vi "Actor Core.vi"(8 "error in":errorcluster, 11 "Nested in":refnum<class "UI Actor.lvclass">) -> (0 "error out":errorcluster, 3 "Actor out":refnum<class "Actor.lvclass">)   [LabVIEW 2020, in "UI Actor.lvlib" / "UI Actor.lvclass"]
doc: "Override de Actor Core, nos sirve para crear una interfaz amigable con el usuario."
uses:
  UI Actor.lvclass
  C:/Program Files/National Instruments/LabVIEW 2020/vi.lib/ActorFramework/Actor/Actor.lvclass
  <vilib>/ActorFramework/Actor/Actor.lvclass
  <vilib>/ActorFramework/Actor/Actor.lvclass/Actor.ctl
  <vilib>/ActorFramework/Message Enqueuer/Message Enqueuer.lvclass/Message Enqueuer.ctl
  UI Actor.lvclass/UI Actor.ctl
  <vilib>/ActorFramework/Message Enqueuer/Init from Existing Queue.vi
  <vilib>/ActorFramework/Message Enqueuer/Enqueue.vi
  UI Actor Messages/Close VISA Msg/Close VISA Msg.lvclass
  C:/Program Files/National Instruments/LabVIEW 2020/vi.lib/ActorFramework/Message/Message.lvclass
  <vilib>/ActorFramework/Stop Msg/Stop Msg.lvclass
  <vilib>/ActorFramework/Message Priority Queue/Priority Enqueue.vi
  <vilib>/ActorFramework/Message Enqueuer/Message Enqueuer.lvclass
  Abstract/Serial Device/Serial Device.lvclass
panel:
  out "String":string
  in  "Channel":u8
  out "Distancia":i32(slide) scale=0.0..200.0
  in  "CANAL2":bool
  in  "CANAL1 3":bool
  in  "Pin Number":u8
  in  "Set Pin":bool
  in  "CANAL1 2":bool
  in  "Set Port":bool[](array[boolean])
  in  "CANAL1 5":bool
  in  "Pin Number":u8
  out "Read Pin":bool
  in  "CANAL1 4":bool
  out "Read Port":bool[](array[boolean])
  # "Pin del 1 al 4"
  # "MSB"
  # "LSB"
  # "Pin del 1 al 4"
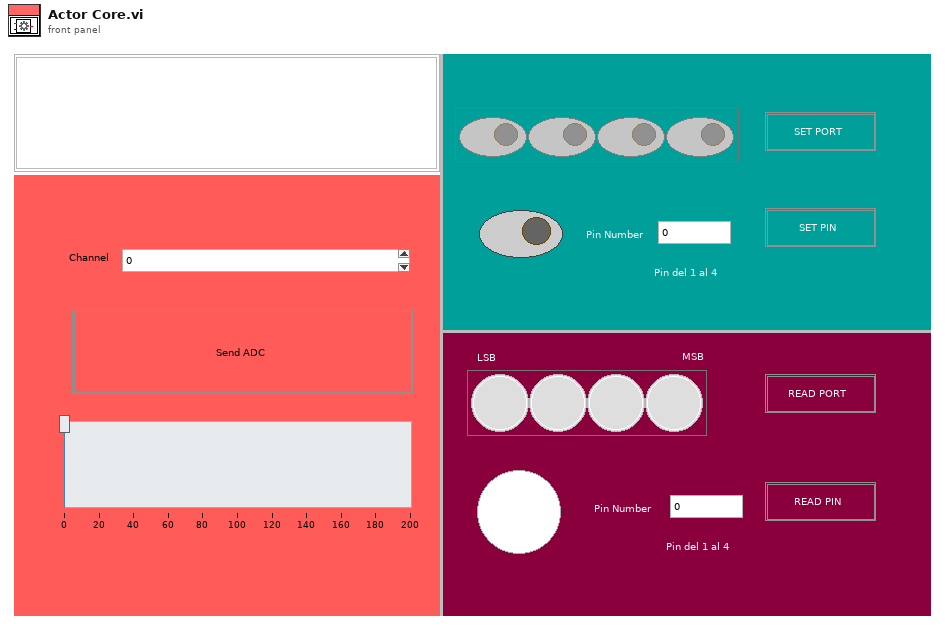
[diagram p1: front panel]
types:
  T1 = cluster{"Stop":refnum<user-event>, "LIGHT":refnum<user-event>, "Distancia":refnum<user-event>, "Read Port":refnum<user-event>, "Read Pin":refnum<user-event>, "String":refnum<user-event>}
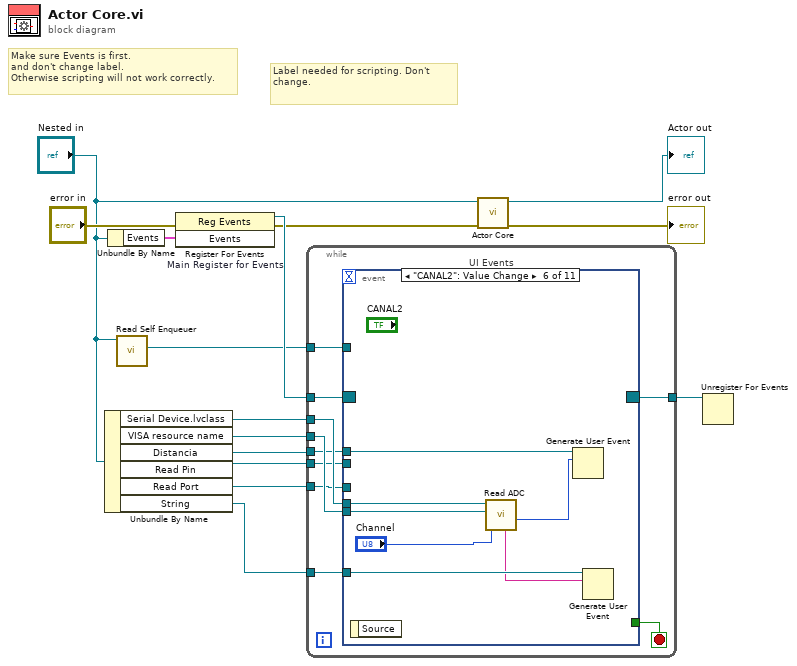
[diagram p0: block diagram]
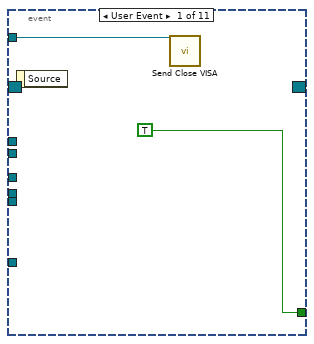
[diagram p2: hidden frame]
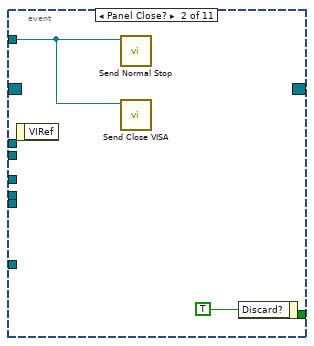
[diagram p3: hidden frame]
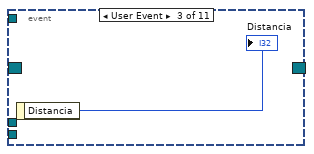
[diagram p4: hidden frame]
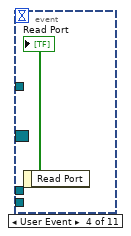
[diagram p5: hidden frame]
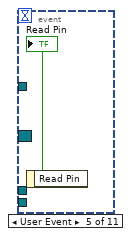
[diagram p6: hidden frame]
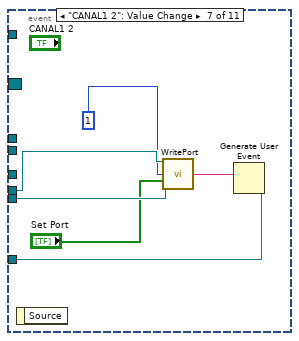
[diagram p7: hidden frame]
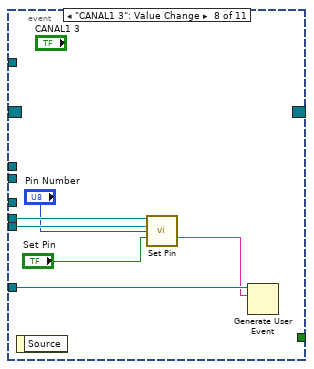
[diagram p8: hidden frame]
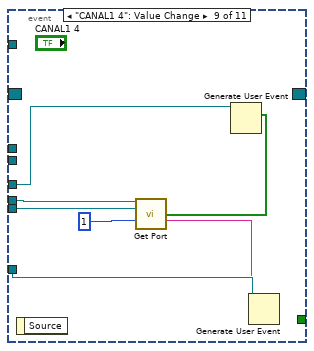
[diagram p9: hidden frame]
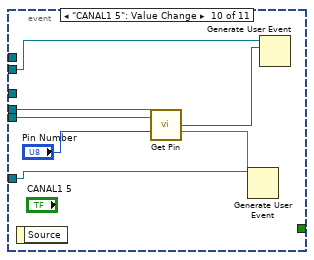
[diagram p10: hidden frame]
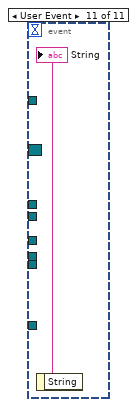
[diagram p11: hidden frame]
diagram:
  # "Label needed for scripting. Don't change."
  # "Make sure Events is first.\nand don't change label.\nOtherwise scripting will not work correctly."
  n1 = Unbundle By Name("Nested in") -> ("Serial Device.lvclass"=w6:refnum<class "Serial Device.lvclass">, "VISA resource name"=w5:refnum<visa-resource-name>, "Distancia"=w4:refnum<user-event>, "Read Pin"=w2:refnum<user-event>, "Read Port"=w3:refnum<user-event>, "String"=w1:refnum<user-event>)
  n2 = Unbundle By Name("Nested in") -> ("Events"=w12:T1)
  n3 = call <vilib>:"Read Self Enqueuer.vi"("Actor"="Nested in") -> ("Self Enqueuer"=w10:refnum<class "Message Enqueuer.lvclass">)  [unwired: 10 in]
  n4 = register-events "Main Register for Events"(error in="error in", w12) -> (reference out=w13:refnum<event-registration>, error out=w8:errorcluster)  [unwired: 1 in]
  n5 = while {
    tunnel: w13 -> [w25]
    tunnel: [w23] -> w11
    tunnel: w10 -> [w22]
    tunnel: w6 -> [w21]
    tunnel: w5 -> [w20]
    tunnel: w4 -> [w19]
    tunnel: w1 -> [w18]
    tunnel: w3 -> [w17]
    tunnel: w2 -> [w16]
    stop <- w24 stop-if-true
    n6 = event "UI Events" shown="[5] \"CANAL2\": Value Change" {
      selector: w25 -> [_ _ _ _ _ _ _ _ _ _ _]
      dyn-events: [_ _ _ _ _ _ _ _ _ _ _] -> w23
      timeout: _ -> [_ _ _ _ _ _ _ _ _ _ _]
      tunnel: [TRUE _ _ _ _ _ _ _ _ _ _] -> w24
      tunnel: w22 -> [w26 w28 _ _ _ _ _ _ _ _ _]
      tunnel: w21 -> [_ _ _ _ _ w39 w45 w51 w58 w65 _]
      tunnel: w20 -> [_ _ _ _ _ w38 w44 w50 w57 w64 _]
      tunnel: w19 -> [_ _ _ _ _ w36 _ _ _ _ _]
      tunnel: w18 -> [_ _ _ _ _ w34 w42 w47 w53 w60 _]
      tunnel: w17 -> [_ _ _ _ _ _ _ _ w55 _ _]
      tunnel: w16 -> [_ _ _ _ _ _ _ _ _ w62 _]
      event User Event {
        n7 = event-data() -> ()  [unwired: 1 in, 1 out]
        n8 = call "Send Close VISA.vi"("Message Enqueuer"=w26) -> ()  [unwired: 9 in, 2 out]
      }
      event Panel Close? {
        n9 = event-data() -> ()  [unwired: 1 in, 1 out]
        n10 = call <vilib>:"Send Normal Stop.vi"("Message Enqueuer"=w28) -> ()  [unwired: 10 in, 1 out]
        n11 = call "Send Close VISA.vi"("Message Enqueuer"=w28) -> ()  [unwired: 9 in, 2 out]
        n12 = event-data("Discard?"=TRUE) -> ()  [unwired: 1 in, 1 out]
      }
      event User Event {
        n13 = event-data() -> ("Distancia"=→"Distancia":i32)  [unwired: 1 in]
      }
      event User Event {
        n14 = event-data() -> ("Read Port"=→"Read Port":bool[])  [unwired: 1 in]
      }
      event User Event {
        n15 = event-data() -> ("Read Pin"=→"Read Pin":bool)  [unwired: 1 in]
      }
      event "CANAL2": Value Change {
        n16 = event-data() -> ()  [unwired: 1 in, 1 out]
        n17 = call-dynamic "Read ADC.vi"("Canal"="Channel", "VISA resource name"=w38, "Serial Device in"=w39) -> ("Response"=w35:i32, "String"=w33:string)  [unwired: 4 in, 3 out]
        n18 = Generate User Event(user event=w36, event data cluster=w35) -> ()  [unwired: 2 in, 2 out]
        n19 = Generate User Event(user event=w34, event data cluster=w33) -> ()  [unwired: 2 in, 2 out]
      }
      event "CANAL1 2": Value Change {
        n20 = event-data() -> ()  [unwired: 1 in, 1 out]
        n21 = call-dynamic "WritePort.vi"("Serial Device in"=w45, "VISA resource name"=w44, "Puerto"=u8 1, "Array"="Set Port") -> ("Expected response"=w41:string)  [unwired: 8 in, 3 out]
        n22 = Generate User Event(user event=w42, event data cluster=w41) -> ()  [unwired: 2 in, 2 out]
      }
      event "CANAL1 3": Value Change {
        n23 = event-data() -> ()  [unwired: 1 in, 1 out]
        n24 = call-dynamic "Set Pin.vi"("Serial Device in"=w51, "VISA resource name"=w50, "Pin"="Pin Number", "Pin State"="Set Pin") -> ("Response"=w46:string)  [unwired: 8 in, 3 out]
        n25 = Generate User Event(user event=w47, event data cluster=w46) -> ()  [unwired: 2 in, 2 out]
      }
      event "CANAL1 4": Value Change {
        n26 = event-data() -> ()  [unwired: 1 in, 1 out]
        n27 = call-dynamic "Get Port.vi"("Serial Device in"=w58, "VISA resource name"=w57, "Puerto"=u8 1) -> ("bool response"=w54:bool[], "Response"=w52:string)  [unwired: 8 in, 3 out]
        n28 = Generate User Event(user event=w55, event data cluster=w54) -> ()  [unwired: 2 in, 2 out]
        n29 = Generate User Event(user event=w53, event data cluster=w52) -> ()  [unwired: 2 in, 2 out]
      }
      event "CANAL1 5": Value Change {
        n30 = event-data() -> ()  [unwired: 1 in, 1 out]
        n31 = call-dynamic "Get Pin.vi"("Serial Device in"=w65, "VISA resource name"=w64, "Pin"="Pin Number") -> ("Boolean"=w61:bool, "Response"=w59:string)  [unwired: 8 in, 3 out]
        n32 = Generate User Event(user event=w60, event data cluster=w59) -> ()  [unwired: 2 in, 2 out]
        n33 = Generate User Event(user event=w62, event data cluster=w61) -> ()  [unwired: 2 in, 2 out]
      }
      event User Event {
        n34 = event-data() -> ("String"=→"String":string)  [unwired: 1 in]
      }
    }
  }
  n35 = call-parent "Actor Core.vi"("error in"=w8, "Actor in"="Nested in") -> ("error out"=→"error out":errorcluster, "Actor out"=→"Actor out":refnum<class "Actor.lvclass">)  [unwired: 8 in]
  n36 = Unregister For Events(event registration refnum=w11) -> ()  [unwired: 1 in, 1 out]
